vi "Get Factors.vi"(11 "Number to Factor":u64) -> (3 "Factors":u64[](array[numeric]))   [LabVIEW 2013, in "Problem 12.lvlib"]
uses:
  Problem 12.lvlib
  Problem 3/Problem 3.lvlib
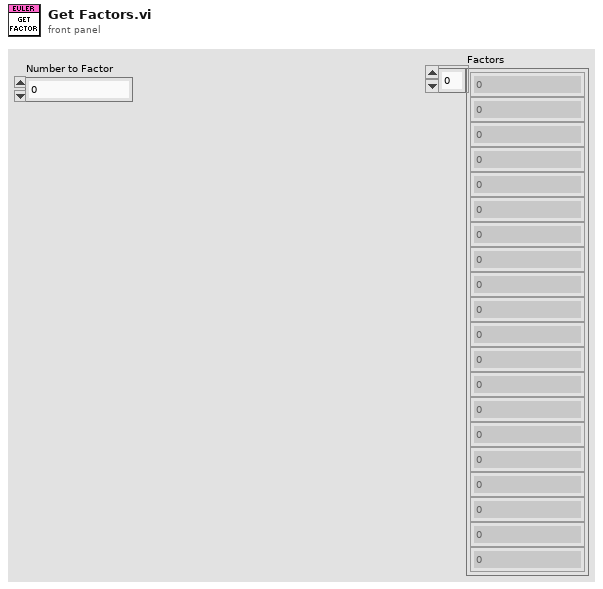
[diagram p1: front panel]
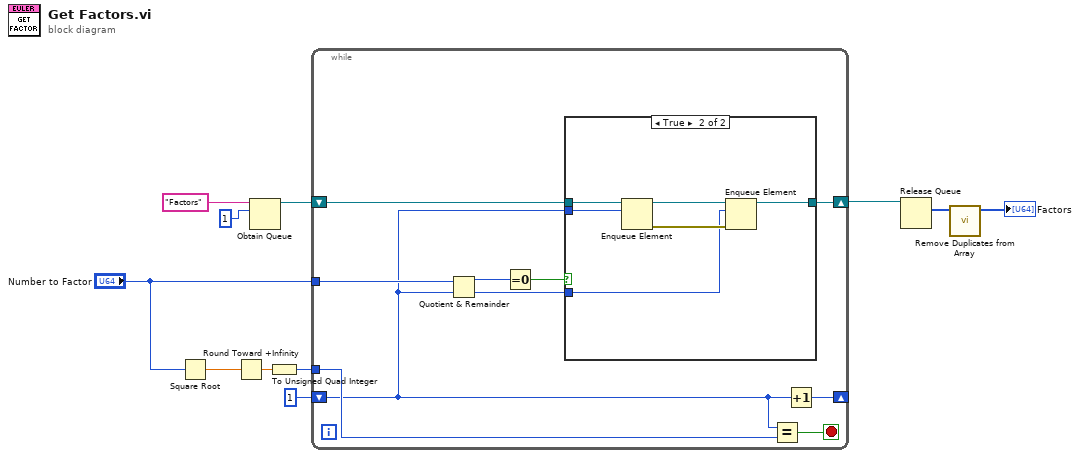
[diagram p0: block diagram]
diagram:
  n1 = Square Root(x="Number to Factor") -> (sqrt(x)=w11:dbl)
  n2 = Round Toward +Infinity(x=w11) -> (ceil(x): smallest int >= x=w10:dbl)
  n3 = Obtain Queue(name (unnamed)="Factors", element data type=u64 1) -> (queue out=w4:refnum<queue>)  [unwired: 3 in, 2 out]
  n4 = To Unsigned Quad Integer(1:w10) -> (0:w8:u64)
  n5 = while {
    tunnel: w8 -> [w19]
    shift-right: [w21] -> _
    shift-left: u64 1 -> [w12]
    tunnel: "Number to Factor" -> [w18]
    shift-right: [w13] -> w3
    shift-left: w4 -> [w14]
    stop <- w20 stop-if-true
    n6 = Quotient & Remainder(x=w18, y=w12) -> (x-y*floor(x/y)=w15:u64, floor(x/y)=w16:u64)
    n7 = Equal To 0?(x=w15) -> (x = 0?=w17:bool)
    n8 = case shown="True" w17 {
      tunnel: w16 -> [_ w25]
      tunnel: w14 -> [w22 w28]
      tunnel: [w22 w24] -> w13
      tunnel: w12 -> [_ w23]
      frame False {
      }
      frame True {
        n9 = Enqueue Element(queue=w28, element=w23) -> (queue out=w27:refnum<queue>, error out=w26:errorcluster)  [unwired: 2 in, 1 out]
        n10 = Enqueue Element(queue=w27, element=w25, error in (no error)=w26) -> (queue out=w24:refnum<queue>)  [unwired: 1 in, 2 out]
      }
    }
    n11 = Equal?(x=w12, y=w19) -> (x = y?=w20:bool)
    n12 = Increment(x=w12) -> (x+1=w21:u64)
  }
  n13 = Release Queue(queue=w3) -> (remaining elements=w2:u64[])  [unwired: 2 in, 2 out]
  n14 = call "Remove Duplicates from Array.vi"("Array with Duplicates"=w2) -> ("Cleaned Array"=→"Factors":u64[])  [unwired: 10 in]
